vi "Load Picture from File.vi"(4 "error in (no error)":errorcluster, 6 "Dialog? (f)":bool, 7 "Path (Empty Path)":path) -> (0 "error out":errorcluster, 2 "Size":cluster{"width":i32, "height":i32}, 3 "Picture":picture)   [LabVIEW 2011]
doc: "Loads a picture file (*.jpg, *.bmp, *.png types supported) into a picture indicator. If Path not wired or Not a Path or empty path, then global ROOT\\Pics\\ folder is searched. Otherwise, Path\\Pics\\ folder is searched."
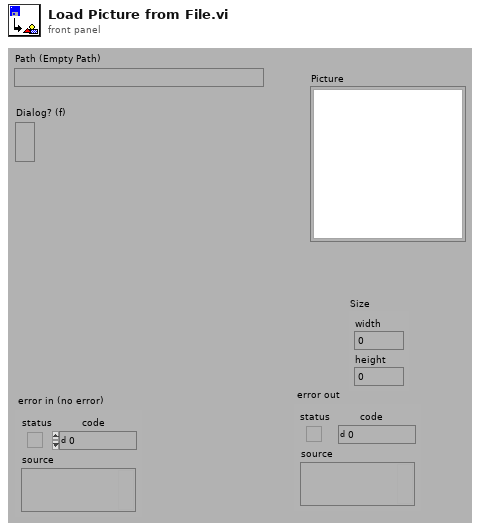
[diagram p1: front panel]
types:
  T1 = typedef "imagedata.ctl" = cluster{"image type":i32, "image depth":i32, "image":u8[], "mask":u8[], "colors":u32[], "Rectangle":cluster{"left":i16, "top":i16, "right":i16, "bottom":i16}}
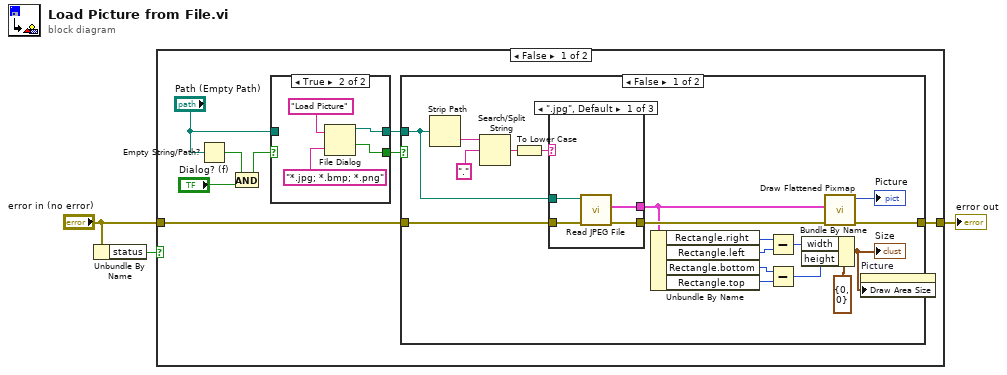
[diagram p0: block diagram]
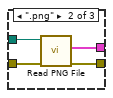
[diagram p2: hidden frame]
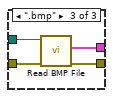
[diagram p3: hidden frame]
diagram:
  n1 = Unbundle By Name("error in (no error)") -> ("status"=w1:bool)
  n2 = case shown="False" w1 {
    tunnel: "error in (no error)" -> [w11 w48]
    tunnel: [w10 w48] -> w3
    frame False {
      n3 = Empty String/Path?(string/path="Path (Empty Path)") -> (empty?=w5:bool)
      n4 = And(x=w5, y="Dialog? (f)") -> (x .and. y?=w4:bool)
      n5 = case shown="True" w4 {
        selector: w4 -> [w42 _]
        tunnel: [w43 w47] -> w9
        tunnel: "Path (Empty Path)" -> [w43 _]
        tunnel: [w42 w44] -> w7
        frame False {
        }
        frame True {
          n6 = File Dialog(6:"*.jpg; *.bmp; *.png", 7:"Load Picture") -> (1:w44:bool, 3:w47:path)  [unwired: 1 in, 6 out]
        }
      }
      n7 = case shown="False" w7 {
        tunnel: w11 -> [w28 w41]
        tunnel: [w27 w41] -> w10
        tunnel: w9 -> [w26 _]
        frame False {
          n8 = Strip Path(path=w26) -> (name=w25:string)  [unwired: 1 out]
          n9 = Search/Split String(string=w25, search string/char (-)=".") -> (match + rest of string=w23:string)  [unwired: 3 out]
          n10 = To Lower Case(string=w23) -> (all lower case string=w22:string)
          n11 = case shown="\".jpg\", Default" w22 {
            tunnel: w26 -> [w32 w35 w39]
            tunnel: w28 -> [w31 w36 w40]
            tunnel: [w30 w34 w38] -> w27
            tunnel: [w29 w33 w37] -> w19
            frame ".jpg", Default {
              n12 = call <vilib>:"Read JPEG File.vi"("error in (no error)"=w31, "path to JPEG file"=w32) -> ("error out"=w30:errorcluster, "image data"=w29:T1)  [unwired: 8 out]
            }
            frame ".png" {
              n13 = call <vilib>:"Read PNG File.vi"("error in (no error)"=w36, "path to PNG file"=w35) -> ("error out"=w34:errorcluster, "image data"=w33:T1)  [unwired: 8 out]
            }
            frame ".bmp" {
              n14 = call <vilib>:"Read BMP File.vi"("error in (no error)"=w40, "path to BMP file"=w39) -> ("error out"=w38:errorcluster, "image data"=w37:T1)  [unwired: 8 out]
            }
          }
          n15 = Unbundle By Name(w19) -> ("Rectangle.right"=w18:i16, "Rectangle.left"=w17:i16, "Rectangle.bottom"=w15:i16, "Rectangle.top"=w14:i16)
          n16 = Subtract(x=w18, y=w17) -> (x-y=w16:i16)
          n17 = Subtract(x=w15, y=w14) -> (x-y=w13:i16)
          n18 = Bundle By Name(cluster=cluster{"width":i32, "height":i32} {"width"=0, "height"=0} ("Size"), "width"=w16, "height"=w13) -> (w12:cluster{"width":i32, "height":i32})
          "Size" <- w12
          n19 = call <vilib>:"Draw Flattened Pixmap.vi"("image data"=w19) -> ("new picture"=→"Picture":picture)  [unwired: 1 in, 7 out]
          n20 = property on="Picture" class="Pict"("Draw Area Size"=w12) -> ()  [unwired: 2 in, 2 out]
        }
        frame True {
        }
      }
    }
    frame True {
    }
  }
  "error out" <- w3
